vi "TrajectoryExecuteRelative.vi"(8 "Init":bool, 10 "End Relative\nOrientation Deg":dbl, 11 "Trajectory":T1 {"States"."POSE"."ROTATION"."SIN" format="%13.4f"; "States"."POSE"."ROTATION"."COS" format="%13.4f"; "States"."POSE"."ROTATION"."VALUE" format="%13.4f"; "States"."POSE"."TRANSLATION"."Y" format="%14.3f"; "States"."POSE"."TRANSLATION"."X" format="%14.3f"; "TotalTImeSecs" format="%20.3f"}) -> (0 "AtReference":bool, 2 "Done":bool, 3 "Chassis Velocity Target Met,Met,Rad":T6 {"vOmega" format="%10.3f"; "vY" format="%10.3f"; "vX" format="%10.3f"})   [LabVIEW 2023]
uses:
  <vilib>/Rock Robotics/WPI/ThirdParty/JAS_Junk/TrajLib/Trajectory_Library.lvlib
  TrajectoryGlobals.vi
  <vilib>/Rock Robotics/WPI/ThirdParty/JAS_Junk/TrajLib/TypeDef/CHASSIS_SPEEDS.ctl
  <vilib>/Rock Robotics/WPI/ThirdParty/JAS_Junk/TrajLib/TypeDef/TRANSLATION2D.ctl
  <vilib>/Rock Robotics/WPI/ThirdParty/JAS_Junk/TrajLib/TypeDef/ROTATION2D.ctl
  <vilib>/Rock Robotics/WPI/ThirdParty/JAS_Junk/TrajLib/TypeDef/POSE2D.ctl
  <vilib>/Rock Robotics/WPI/ThirdParty/JAS_Junk/TrajLib/TypeDef/TRAJ_STATE.ctl
  <vilib>/Rock Robotics/WPI/ThirdParty/JAS_Junk/TrajLib/TypeDef/TRAJECTORY.ctl
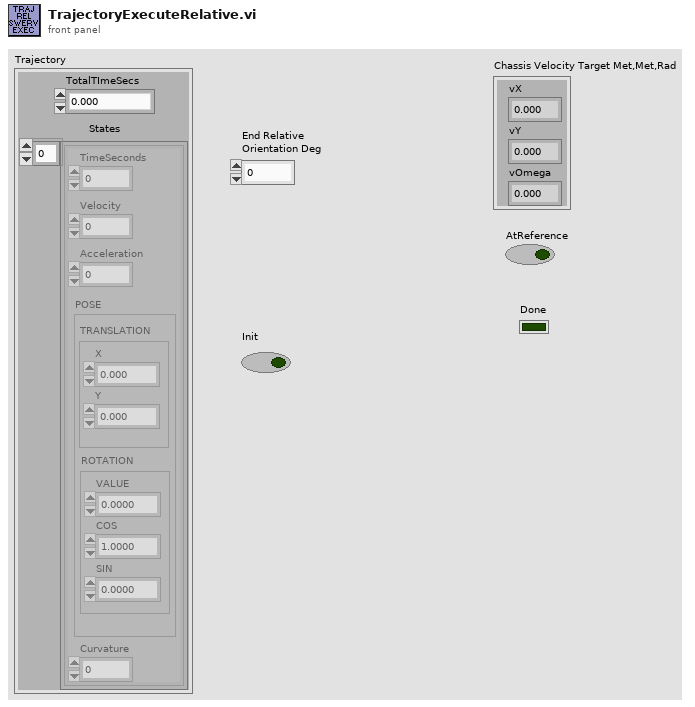
[diagram p1: front panel]
types:
  T1 = typedef "Trajectory_Library.lvlib/TRAJECTORY.ctl" = cluster{"TotalTImeSecs":dbl, "States":T2[]}
  T2 = typedef "Trajectory_Library.lvlib/TRAJ_STATE.ctl" = cluster{"TimeSeconds":dbl, "Velocity":dbl, "Acceleration":dbl, "POSE":T3, "Curvature":dbl}
  T3 = typedef "Trajectory_Library.lvlib/POSE2D.ctl" = cluster{"TRANSLATION":T4, "ROTATION":T5}
  T4 = typedef "Trajectory_Library.lvlib/TRANSLATION2D.ctl" = cluster{"X":dbl, "Y":dbl}
  T5 = typedef "Trajectory_Library.lvlib/ROTATION2D.ctl" = cluster{"VALUE":dbl, "COS":dbl, "SIN":dbl}
  T6 = typedef "Trajectory_Library.lvlib/CHASSIS_SPEEDS.ctl" = cluster{"vX":dbl, "vY":dbl, "vOmega":dbl}
  T7 = typedef "Trajectory_Library.lvlib/SWERVE_DRIVE_MODULE_POSITION.ctl" = cluster{"Distance":dbl, "Angle":T5, "P":bool}
  T8 = typedef "Trajectory_Library.lvlib/SWERVE_DRIVE_KINEMATICS.ctl" = cluster{"NumModules":i32, "InverseKinematics":T9, "ForwardKinematics":T9, "Modules":T4[], "PrevCoR":T4, "SavedModuleStates":T10[]}
  T9 = typedef "NI_Matrix.lvlib/RealMatrix.ctl" = dbl[][]
  T10 = typedef "Trajectory_Library.lvlib/SWERVE_DRIVE_MODULE_STATE.ctl" = cluster{"Speed":dbl, "Angle":T5}
  T11 = typedef "Trajectory_Library.lvlib/PID_TUNING.ctl" = cluster{"Kp":dbl, "Ki":dbl, "Kd":dbl, "MaximumIntegral":dbl, "MinimumIntegral":dbl, "IntegralZone":dbl}
  T12 = typedef "Trajectory_Library.lvlib/PROFILED_PID_CONTROLLER.ctl" = cluster{"Controller":T13, "Goal":T14, "Setpoint":T14, "Constraint":T15}
  T13 = typedef "Trajectory_Library.lvlib/PID_CONTROLLER.ctl" = cluster{"Kp":dbl, "Ki":dbl, "Kd":dbl, "Period":dbl, "Max_Integral":dbl, "Min_Integral":dbl, "Max_Input":dbl, "Min_Input":dbl, "Continuous":bool, "PositionError":dbl, "VelocityError":dbl, "PrevError":dbl, "Total_Integral":dbl, "PositionTolerance":dbl, "VelocityTolerance":dbl, "SetPoint":dbl, "Kf":dbl, "Prev_Deriv":dbl, "Prev_Deriv 2":dbl, "DerivativeFilter":bool, "Min_Output":dbl, "Max_Output":dbl, "Prev_F_P":dbl, "Prev_F_P_2":dbl, "AntiWindupActive":bool, "Measurement":dbl, "IntegralZone":dbl}
  T14 = typedef "Trajectory_Library.lvlib/TRAPEZOID_PROFILE_STATE.ctl" = cluster{"Position":dbl, "Velocity":dbl}
  T15 = typedef "Trajectory_Library.lvlib/TRAPEZOID_PROFILE_CONSTRAINT.ctl" = cluster{"MaxVelocity":dbl, "MaxAcceleration":dbl}
  T16 = typedef "Trajectory_Library.lvlib/HOLONOMIC_PACK_TUNING.ctl" = cluster{"X PID Tuning":T11, "Y PID Tuning":T11, "thetaProfiledPID_CTRL":T12}
  T17 = typedef "Trajectory_Library.lvlib/HOLONOMIC_DRV_CTRL.ctl" = cluster{"poseTolerance":T3, "poseError":T3, "Enabled":bool, "PID_xCtrl":T13, "PID_yCtrl":T13, "PROF_PID_thetaCtrl":T12, "RotationError":T5, "FirstRun":bool}
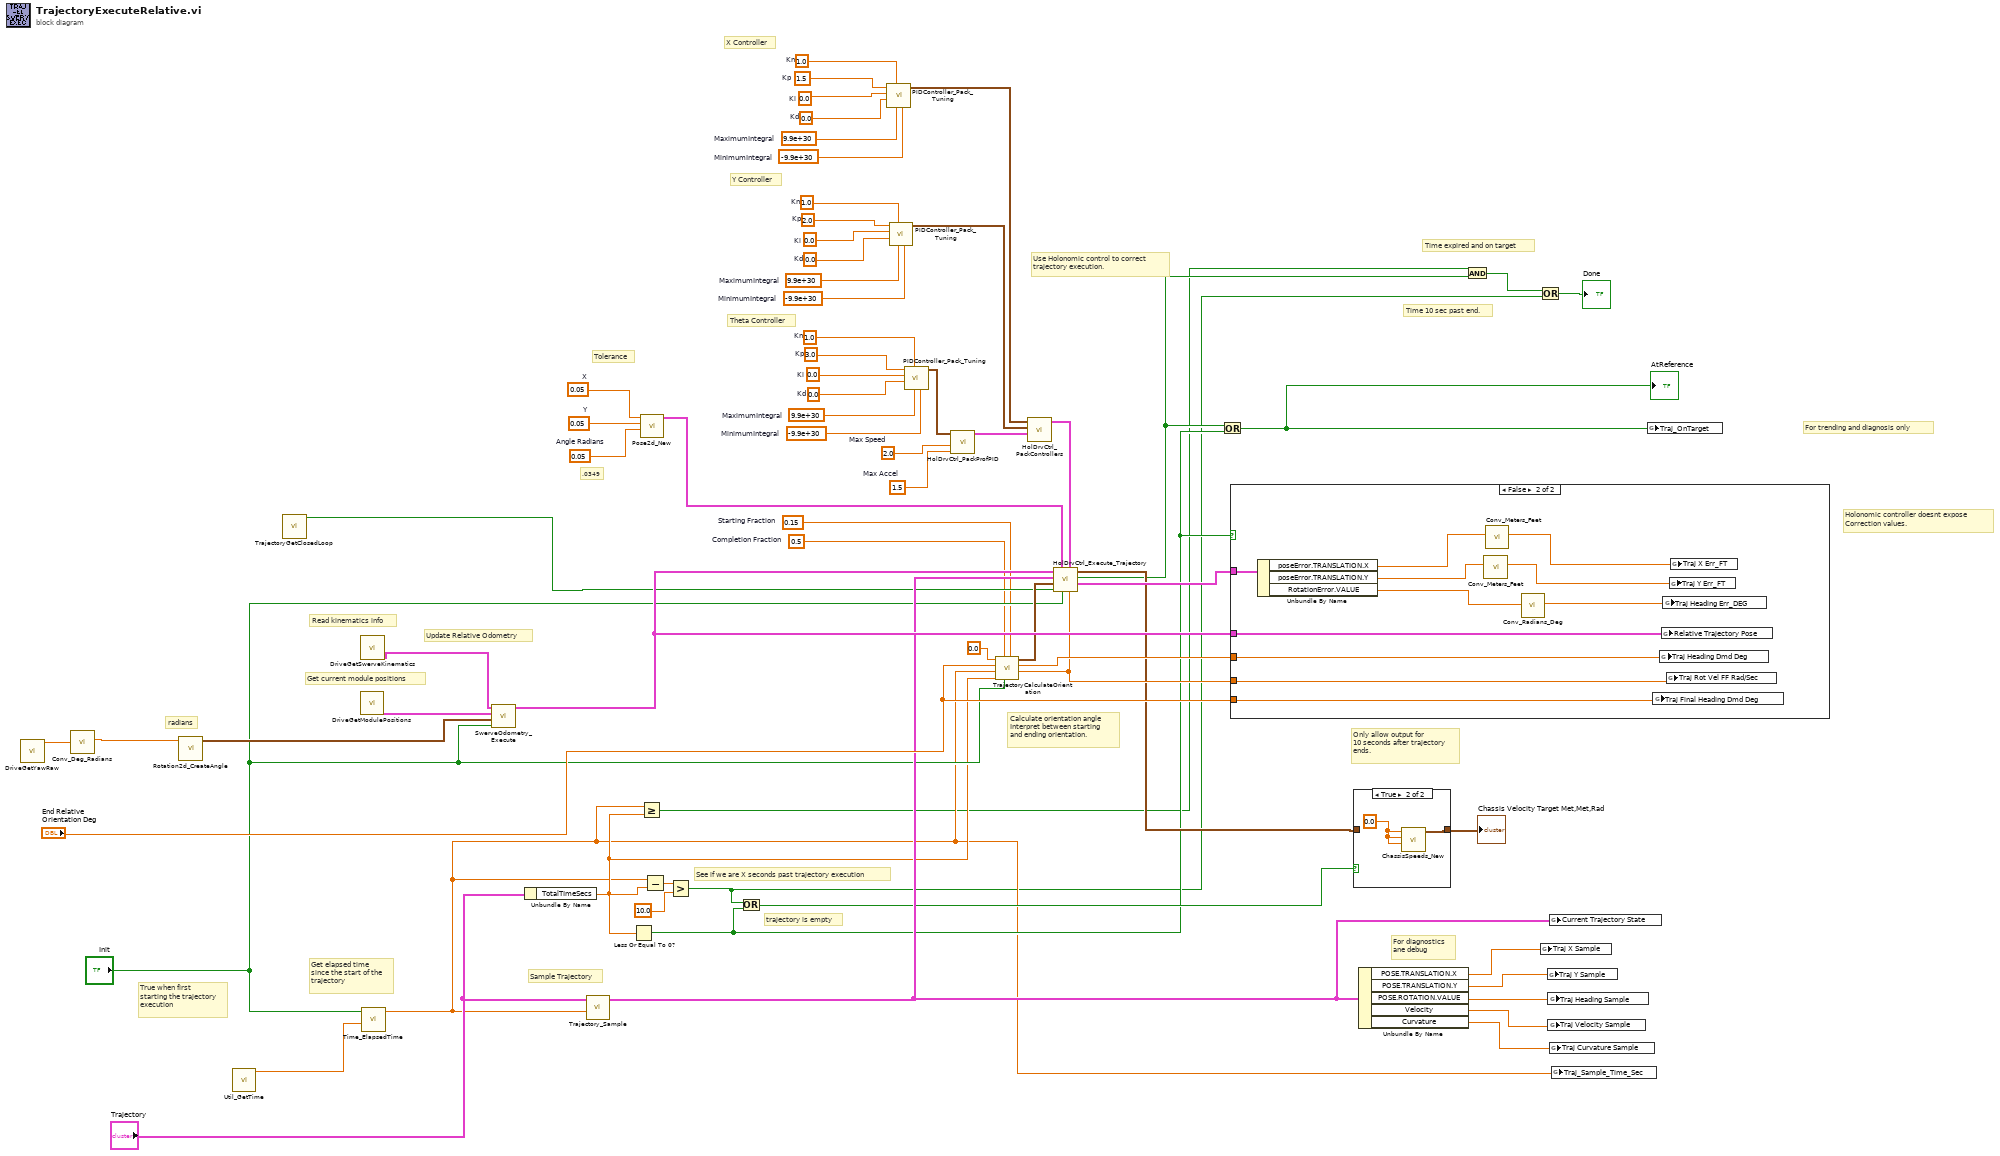
[diagram p0: block diagram]
diagram:
  w3 = 0.05  # X
  w2 = 0.05  # Y
  w4 = 0.05  # Angle Radians
  w5 = 0.15  # Starting Fraction
  w6 = 0.5  # Completion Fraction
  w17 = 1.5  # Max Accel
  w18 = 2.0  # Max Speed
  w36 = 1.0  # Kn
  w39 = 3.0  # Kp
  w48 = 0.0  # Ki
  w49 = 0.0  # Kd
  w50 = 9.9e+30  # MaximumIntegral
  w51 = -9.9e+30  # MinimumIntegral
  w34 = 1.0  # Kn
  w37 = 1.5  # Kp
  w40 = 0.0  # Ki
  w41 = 0.0  # Kd
  w42 = 9.9e+30  # MaximumIntegral
  w43 = -9.9e+30  # MinimumIntegral
  w35 = 1.0  # Kn
  w38 = 2.0  # Kp
  w44 = 0.0  # Ki
  w45 = 0.0  # Kd
  w46 = 9.9e+30  # MaximumIntegral
  w47 = -9.9e+30  # MinimumIntegral
  # ".0349"
  # "Tolerance"
  # "Time 10 sec past end."
  # "Time expired and on target"
  # "trajectory is empty"
  # "Theta Controller"
  # "Y Controller"
  # "X Controller"
  # "Calculate orientation angle\nInterpret between starting\nand ending orientation."
  # "Get current module positions"
  # "True when first\nstarting the trajectory\nexecution"
  # "Get elapsed time\nsince the start of the\ntrajectory"
  # "Holonomic controller doesnt expose\nCorrection values."
  # "Use Holonomic control to correct\ntrajectory execution."
  # "For trending and diagnosis only"
  # "For diagnostics\nane debug"
  # "Update Relative Odometry"
  # "Read kinematics info"
  # "Sample Trajectory"
  # "See if we are X seconds past trajectory execution"
  # "radians"
  # "Only allow output for\n10 seconds after trajectory\nends."
  n1 = call "DriveGetYawRaw.vi"() -> ("YawRaw"=w16:dbl)  [unwired: 11 in]
  n2 = call <vilib>:"Conv_Deg_Radians.vi"("Degress"=w16) -> ("Radians"=w15:dbl)  [unwired: 10 in]
  n3 = call <vilib>:"Rotation2d_CreateAngle.vi"("Angle"=w15) -> ("ROTATION"=w64:T5)  [unwired: 10 in]
  n4 = call <vilib>:"Util_GetTime.vi"() -> ("FPGA_Time_Seconds"=w63:dbl)  [unwired: 9 in, 2 out]
  n5 = call "TrajectoryGetClosedLoop.vi"() -> ("AUTO_CLOSED_LOOP"=w21:bool)  [unwired: 11 in]
  n6 = call "DriveGetModulePositions.vi"() -> ("Swerve_Drive_Modual_Positions"=w19:T7[])  [unwired: 11 in]
  n7 = call "DriveGetSwerveKinematics.vi"() -> ("SWERVE_DRIVE_KINEMATICS"=w20:T8)  [unwired: 11 in]
  n8 = call <vilib>:"Time_ElapsedTime.vi"("PassthroughTime_SEC"=w63, "Reset"="Init") -> ("Elapsed Time Sec"=w12:dbl)  [unwired: 9 in]
  n9 = call <vilib>:"SwerveOdometry_Execute.vi"("Init"="Init", "Rotation"=w64, "Swerve Module Positions"=w19, "SWERVE_DRIVE_KINEMATICS"=w20) -> ("Current Pose"=w32:T3)  [unwired: 5 in, 2 out]
  n10 = Unbundle By Name("Trajectory") -> ("TotalTImeSecs"=w13:dbl)
  n11 = call <vilib>:"Trajectory_Sample.vi"("Time"=w12, "InputTRAJECTORY"="Trajectory") -> ("OutputTRAJ_STATE"=w27:T2)  [unwired: 9 in]
  n12 = Less Or Equal To 0?(x=w13) -> (x <= 0?=w23:bool)
  n13 = Greater Or Equal?(x=w12, y=w13) -> (x >= y?=w8:bool)
  n14 = call <vilib>:"Pose2d_New.vi"("Heading"=w4, "Y"=w2, "X"=w3) -> ("out POSe"=w1:T3)  [unwired: 8 in]
  n15 = Subtract(x=w12, y=w13) -> (x-y=w67:dbl)
  n16 = Greater?(x=w67, y=10.0) -> (0:w7:bool)
  n17 = Or(x=w7, y=w23) -> (x .or. y?=w25:bool)
  n18 = call <vilib>:"PIDController_Pack_Tuning.vi"("MinimumIntegral"=w43, "MaximumIntegral"=w42, "Kn"=w34, "Kd"=w41, "Ki"=w40, "Kp"=w37) -> ("PID Tuning"=w52:T11)  [unwired: 5 in]
  n19 = call <vilib>:"PIDController_Pack_Tuning.vi"("MinimumIntegral"=w47, "MaximumIntegral"=w46, "Kn"=w35, "Kd"=w45, "Ki"=w44, "Kp"=w38) -> ("PID Tuning"=w53:T11)  [unwired: 5 in]
  n20 = call <vilib>:"PIDController_Pack_Tuning.vi"("MinimumIntegral"=w51, "MaximumIntegral"=w50, "Kn"=w36, "Kd"=w49, "Ki"=w48, "Kp"=w39) -> ("PID Tuning"=w33:T11)  [unwired: 5 in]
  n21 = call <vilib>:"HolDrvCtrl_PackProfPID.vi"("Max Accel"=w17, "Max Speed"=w18, "Theta PID Tuning"=w33) -> ("Theta PID CONTROLLER"=w54:T12)  [unwired: 8 in]
  n22 = call "TrajectoryCalculateOrientation.vi"("Starting Fraction"=w5, "Init"="Init", "Completion Fraction"=w6, "Total Trajectory Time Sec"=w13, "Elapsed Traj Time Sec"=w12, "End Orientation Demand DEG"="End Relative\nOrientation Deg", "Starting Orientation  DEG"=0.0) -> ("Rotational Velocity Rad Per Sec"=w29:dbl, "Orientation Demand Deg"=w57:dbl, "Orientation Demand"=w31:T5)  [unwired: 2 in]
  n23 = call <vilib>:"HolDrvCtrl_PackControllers.vi"("thetaProfiledPID_CTRL"=w54, "Y PID Tuning"=w53, "X PID Tuning"=w52) -> ("HOLONOMIC_CTRL_PACK_TUNING"=w55:T16)  [unwired: 8 in]
  n24 = call <vilib>:"HolDrvCtrl_Execute_Trajectory.vi"("Rotational Velocity Feedforward \nRad/Sec"=w29, "HOLONOMIC_CTRL_PACK_TUNING"=w55, "Reset"="Init", "Tolerance"=w1, "Enable"=w21, "angleRef"=w31, "desiredTrajState"=w27, "currentPose"=w32) -> ("outHOLONOMIC_DRV_CTRL"=w30:T17, "AtReference"=w9:bool, "calcChassisSpeed"=w26:T6)  [unwired: 1 in]
  n25 = Or(x=w9, y=w23) -> (x .or. y?=w24:bool)
  "AtReference" <- w24
  n26 = case shown="False" w23 {
    tunnel: w57 -> [_ w78]
    tunnel: "End Relative\nOrientation Deg" -> [_ w77]
    tunnel: w32 -> [_ w71]
    tunnel: w30 -> [_ w70]
    tunnel: w29 -> [_ w69]
    frame True {
    }
    frame False {
      n27 = Unbundle By Name(w70) -> ("poseError.TRANSLATION.X"=w75:dbl, "poseError.TRANSLATION.Y"=w74:dbl, "RotationError.VALUE"=w68:dbl)
      n28 = call <vilib>:"Conv_Meters_Feet.vi"("Meters"=w74) -> ("Feet"=w73:dbl)  [unwired: 10 in]
      n29 = call <vilib>:"Conv_Meters_Feet.vi"("Meters"=w75) -> ("Feet"=w72:dbl)  [unwired: 10 in]
      n30 = call <vilib>:"Conv_Radians_Deg.vi"("Radians"=w68) -> ("Degrees"=w76:dbl)  [unwired: 10 in]
      n31 = global write "TrajectoryGlobals.vi" "Traj Final Heading Dmd Deg"(w77) -> ()
      n32 = global write "TrajectoryGlobals.vi" "Traj Heading Dmd Deg"(w78) -> ()
      n33 = global write "TrajectoryGlobals.vi" "Relative Trajectory Pose"(w71) -> ()
      n34 = global write "TrajectoryGlobals.vi" "Traj Heading Err_DEG"(w76) -> ()
      n35 = global write "TrajectoryGlobals.vi" "Traj Rot Vel FF Rad/Sec"(w69) -> ()
      n36 = global write "TrajectoryGlobals.vi" "Traj Y Err_FT"(w73) -> ()
      n37 = global write "TrajectoryGlobals.vi" "Traj X Err_FT"(w72) -> ()
    }
  }
  n38 = case shown="True" w25 {
    tunnel: w26 -> [w79 _]
    tunnel: [w79 w80] -> w65
    frame False {
    }
    frame True {
      w81 = 0.0 ("vX")
      n39 = call <vilib>:"ChassisSpeeds_New.vi"("vAngular"=w81, "vY"=w81, "vX"=w81) -> ("CHASSIS"=w80:T6)  [unwired: 8 in]
    }
  }
  "Chassis Velocity Target Met,Met,Rad" <- w65
  n40 = Unbundle By Name(w27) -> ("POSE.TRANSLATION.X"=w62:dbl, "POSE.TRANSLATION.Y"=w61:dbl, "POSE.ROTATION.VALUE"=w60:dbl, "Velocity"=w59:dbl, "Curvature"=w58:dbl)
  n41 = And(x=w8, y=w9) -> (x .and. y?=w11:bool)
  n42 = Or(x=w11, y=w7) -> (x .or. y?=→"Done":bool)
  n43 = global write "TrajectoryGlobals.vi" "Traj X Sample"(w62) -> ()
  n44 = global write "TrajectoryGlobals.vi" "Traj Y Sample"(w61) -> ()
  n45 = global write "TrajectoryGlobals.vi" "Traj Heading Sample"(w60) -> ()
  n46 = global write "TrajectoryGlobals.vi" "Traj Velocity Sample"(w59) -> ()
  n47 = global write "TrajectoryGlobals.vi" "Current Trajectory State"(w27) -> ()
  n48 = global write "TrajectoryGlobals.vi" "Traj Curvature Sample"(w58) -> ()
  n49 = global write "TrajectoryGlobals.vi" "Traj_Sample_Time_Sec"(w12) -> ()
  n50 = global write "TrajectoryGlobals.vi" "Traj_OnTarget"(w24) -> ()
